vi "GetLoadFilepath.vi"(8 "error in (no error)":errorcluster, 11 "UI_Interaction_Manager in":refnum<class "UI_Interaction_Manager.lvclass">) -> (0 "error out":errorcluster, 1 "Valid?":bool, 2 "Selected Filepath":path, 3 "UI_Interaction_Manager out":refnum<class "UI_Interaction_Manager.lvclass">)   [LabVIEW 2011, in "UI_Interaction_Manager.lvclass"]
uses:
  UI_Interaction_Manager.lvclass
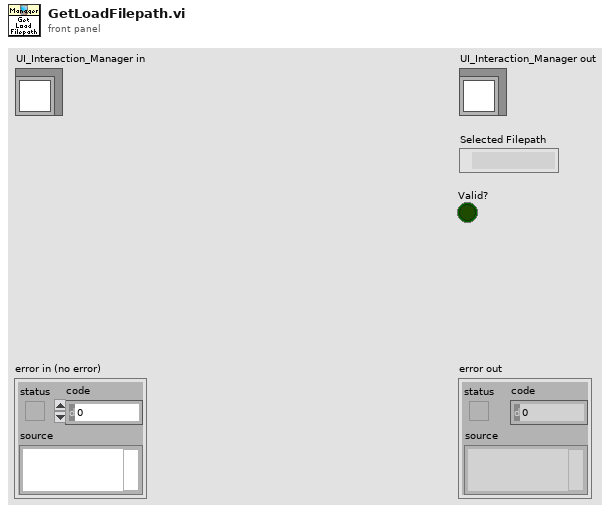
[diagram p1: front panel]
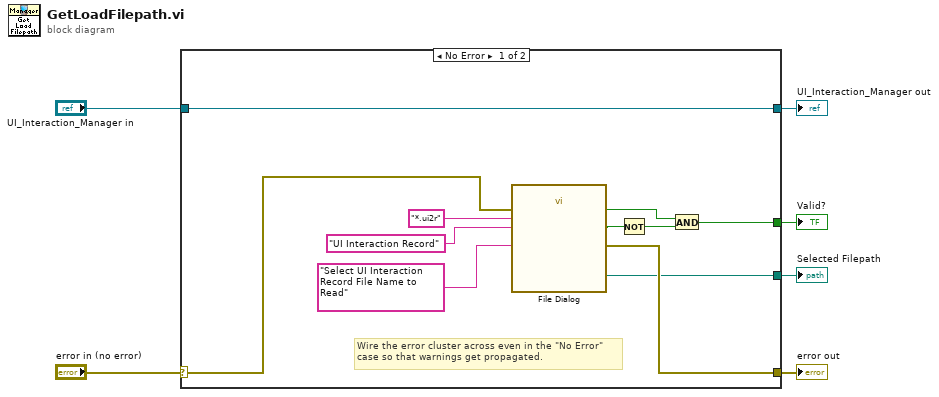
[diagram p0: block diagram]
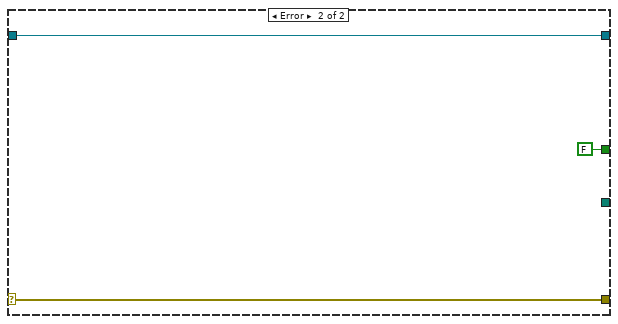
[diagram p2: hidden frame]
diagram:
  n1 = case shown="No Error" "error in (no error)" {
    selector: "error in (no error)" -> [w11 w20]
    tunnel: [w13 w20] -> w3
    tunnel: [w14 w19] -> w4
    tunnel: "UI_Interaction_Manager in" -> [w14 w19]
    tunnel: [w7 FALSE ("cancelled")] -> w2
    tunnel: [w12 _] -> w1
    frame No Error {
      # "Wire the error cluster across even in the \"No Error\"\ncase so that warnings get propagated."
      n2 = call "File Dialog"("prompt"="Select UI Interaction Record File Name to Read", "error in"=w11, "pattern (all files)"="*.ui2r", "pattern label"="UI Interaction Record") -> ("selected path"=w12:path, "exists"=w8:bool, "cancelled"=w10:bool, "error out"=w13:errorcluster)  [unwired: 8 in]
      n3 = Not(x=w10) -> (.not. x?=w9:bool)
      n4 = And(x=w8, y=w9) -> (x .and. y?=w7:bool)
    }
    frame Error {
    }
  }
  "error out" <- w3
  "UI_Interaction_Manager out" <- w4
  "Valid?" <- w2
  "Selected Filepath" <- w1
